vi "Init Graph Parameters.vi"(8 "error in (no error)":errorcluster, 11 "Top Level in":refnum<class "Top Level.lvclass">) -> (0 "error out":errorcluster, 3 "Top Level out":refnum<class "Top Level.lvclass">)   [LabVIEW 2021, in "Top Level.lvlib" / "Top Level.lvclass"]
uses:
  Top Level.lvclass
  Top Level.lvclass/Top Level.ctl
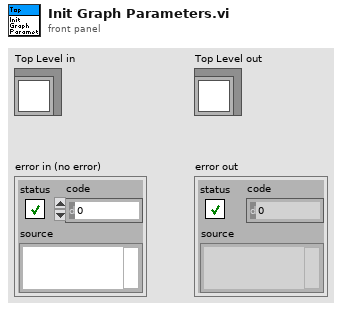
[diagram p1: front panel]
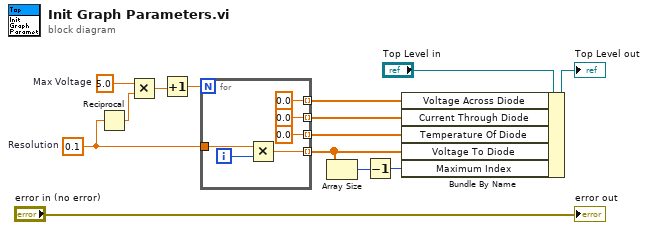
[diagram p0: block diagram]
diagram:
  w10 = 5.0  # Max Voltage
  w9 = 0.1  # Resolution
  n1 = Reciprocal(x=w9) -> (1/x=w11:dbl)
  n2 = Multiply(x=w10, y=w11) -> (x*y=w8:dbl)
  n3 = Increment(x=w8) -> (x+1=w12:dbl)
  n4 = for {
    N: w12 -> [_]
    tunnel: [0.0] -> w4 mode=indexing
    tunnel: w9 -> [w19]
    tunnel: [w17] -> w2 mode=indexing
    tunnel: [0.0] -> w5 mode=indexing
    tunnel: [0.0] -> w3 mode=indexing
    i -> [w18]
    n5 = Multiply(x=w19, y=w18) -> (x*y=w17:dbl)
  }
  n6 = Array Size(array=w2) -> (size(s)=w7:i32)
  n7 = Decrement(x=w7) -> (x-1=w1:i32)
  n8 = Bundle By Name(cluster="Top Level in", "Voltage Across Diode"=w5, "Current Through Diode"=w4, "Temperature Of Diode"=w3, "Voltage To Diode"=w2, "Maximum Index"=w1) -> (→"Top Level out":refnum<class "Top Level.lvclass">)
  "error out" <- "error in (no error)"
